vi "Calc - SGII.vi"(10 "TFFT":dbl, 11 "SG60":dbl) -> (3 "SG11":dbl)   [LabVIEW 2018, in "Controller (Host).lvlib"]
uses:
  Controller (Host).lvlib
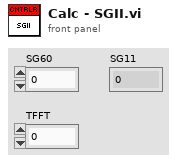
[diagram p1: front panel]
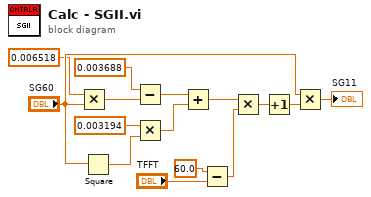
[diagram p0: block diagram]
diagram:
  n1 = Multiply(x=0.006518, y="SG60") -> (x*y=w11:dbl)
  n2 = Square(x="SG60") -> (x^2=w6:dbl)
  n3 = Subtract(x=0.003688, y=w11) -> (x-y=w9:dbl)
  n4 = Multiply(x=0.003194, y=w6) -> (x*y=w7:dbl)
  n5 = Add(x=w9, y=w7) -> (x+y=w5:dbl)
  n6 = Subtract(x=60.0, y="TFFT") -> (x-y=w4:dbl)
  n7 = Multiply(x=w5, y=w4) -> (x*y=w2:dbl)
  n8 = Increment(x=w2) -> (x+1=w1:dbl)
  n9 = Multiply(x="SG60", y=w1) -> (x*y=→"SG11":dbl)
